vi "Combine 2D Affine Transforms.vi"(8 "error in (no error)":errorcluster, 9 "2D Affine Matrix(B)":T1, 11 "2D Affine Matrix (A)":T1) -> (0 "error out":errorcluster, 2 "2D Affine Matrix (A x B)":T1)   [LabVIEW 2020, in "g_ar_toolkit.image.lvlib"]
uses:
  g_ar_toolkit.image.lvlib
  <vilib>/Analysis/Matrix/Datatypes/RealMatrix.ctl
  <vilib>/Analysis/baseanly.llb/Real A x B.vi
  <vilib>/Analysis/NI_AALBase.lvlib
  <vilib>/Analysis/Matrix/NI_Matrix.lvlib
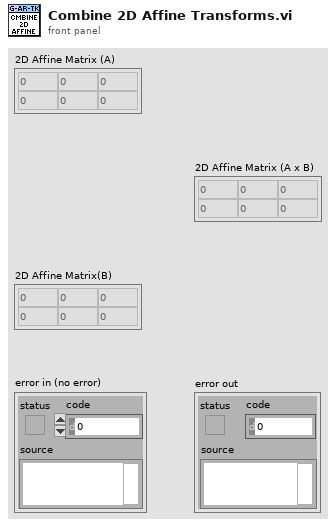
[diagram p1: front panel]
types:
  T1 = typedef "NI_Matrix.lvlib/RealMatrix.ctl" = dbl[][]
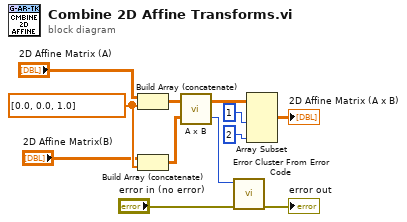
[diagram p0: block diagram]
diagram:
  w12 = dbl[] [0.0, 0.0, 1.0]
  n1 = Build Array (concatenate)("2D Affine Matrix (A)", w12) -> (w11:T1)
  n2 = Build Array (concatenate)("2D Affine Matrix(B)", w12) -> (w10:T1)
  n3 = call-poly <vilib>:"A x B.vi"("B"=w10, "A"=w11) -> ("error"=w4:i32, "A x B"=w9:T1)
  n4 = call <vilib>:"Error Cluster From Error Code.vi"("error in (no error)"="error in (no error)", "error code (0)"=w4) -> ("error out"=→"error out":errorcluster)  [unwired: 7 in]
  n5 = Array Subset(array=w9, length (row)=1 ("row N"), length (col)=2 ("column N")) -> (→"2D Affine Matrix (A x B)":T1)  [unwired: 2 in]
